vi "CropArmPosition.vi"(10 "Position":dbl) -> (2 "New Position":dbl)   [LabVIEW 2015]
uses:
  LowShooter/Implementation/Shooter Global.vi
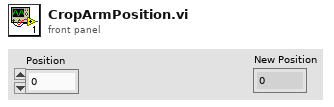
[diagram p1: front panel]
types:
  T1 = typedef "Arm Settings Type Def.ctl" = cluster{"Min Arm Pos":dbl, "Max Arm Pos":dbl, "Drive Pos":dbl, "Ob":dbl}
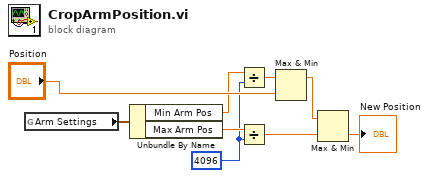
[diagram p0: block diagram]
diagram:
  w1 = 4096
  n1 = global read "Shooter Global.vi" "Arm Settings"() -> (w9:T1)
  n2 = Unbundle By Name(w9) -> ("Min Arm Pos"=w3:dbl, "Max Arm Pos"=w5:dbl)
  n3 = Divide(x=w3, y=w1) -> (x/y=w2:dbl)
  n4 = Divide(x=w5, y=w1) -> (x/y=w4:dbl)
  n5 = Max & Min(x=w2, y="Position") -> (max(x,y)=w7:dbl)  [unwired: 1 out]
  n6 = Max & Min(x=w7, y=w4) -> (min(x,y)=→"New Position":dbl)  [unwired: 1 out]
